vi "TEST_L1_BASELINE.vi"(5 "Serial Number":string="SN_test", 6 "error in":errorcluster, 9 "Instrument VISA in":T1={"AWG VISA"="AgilentGenerator1", "Oscilloscope  VISA "="AgilentOsciloscope", "Integration Board IP"="172.16.17.48", "connection ID"=refnum, "report out"=refnum, "report file path"=path "C:/Users/omartinez/Desktop/L0nL1_Results"}) -> (0 "error out":errorcluster, 3 "VISA Out":T1={"AWG VISA"="AgilentGenerator1", "Oscilloscope  VISA "="AgilentOsciloscope", "Integration Board IP"="172.16.17.48", "connection ID"=refnum, "report out"=refnum, "report file path"=path "C:/Users/omartinez/Desktop/L0nL1_Results"})   [LabVIEW 2012]
uses:
  <vilib>/Utility/NIReport.llb/NI_report.lvclass
  <vilib>/Utility/NIReport.llb/HTML/NI_HTML.lvclass
  <instrlib>/Agilent 8000 Series/Agilent 8000 Series.lvlib
  Sum_Abrilader/L0_Sum_Adder Folder/C/Program Files/National Instruments/LabVIEW 2012/instr.lib/Agilent 81150/Agilent 81150.lvlib
panel:
  out "Current Channel":i32=6
  in  "Combination\n  (Act High)":i32 min=0 max=127 step=1 format="%b"
  in  "Single/Comb":bool=TRUE
  in  "Single Channel Enable":i32(slide) scale=0.0..6.0
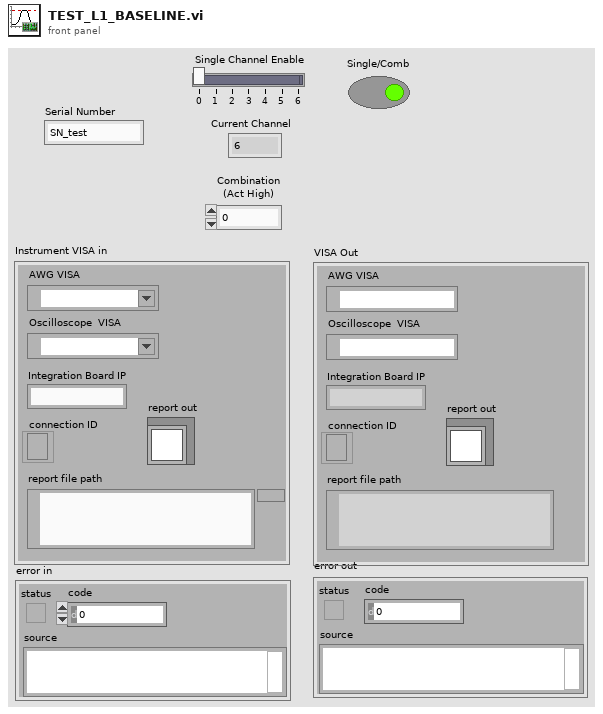
[diagram p1: front panel]
types:
  T1 = cluster{"AWG VISA":refnum<visa-resource-name>, "Oscilloscope  VISA ":refnum<visa-resource-name>, "Integration Board IP":string, "connection ID":refnum<k5>, "report out":refnum<class "NI_report.lvclass">, "report file path":path}
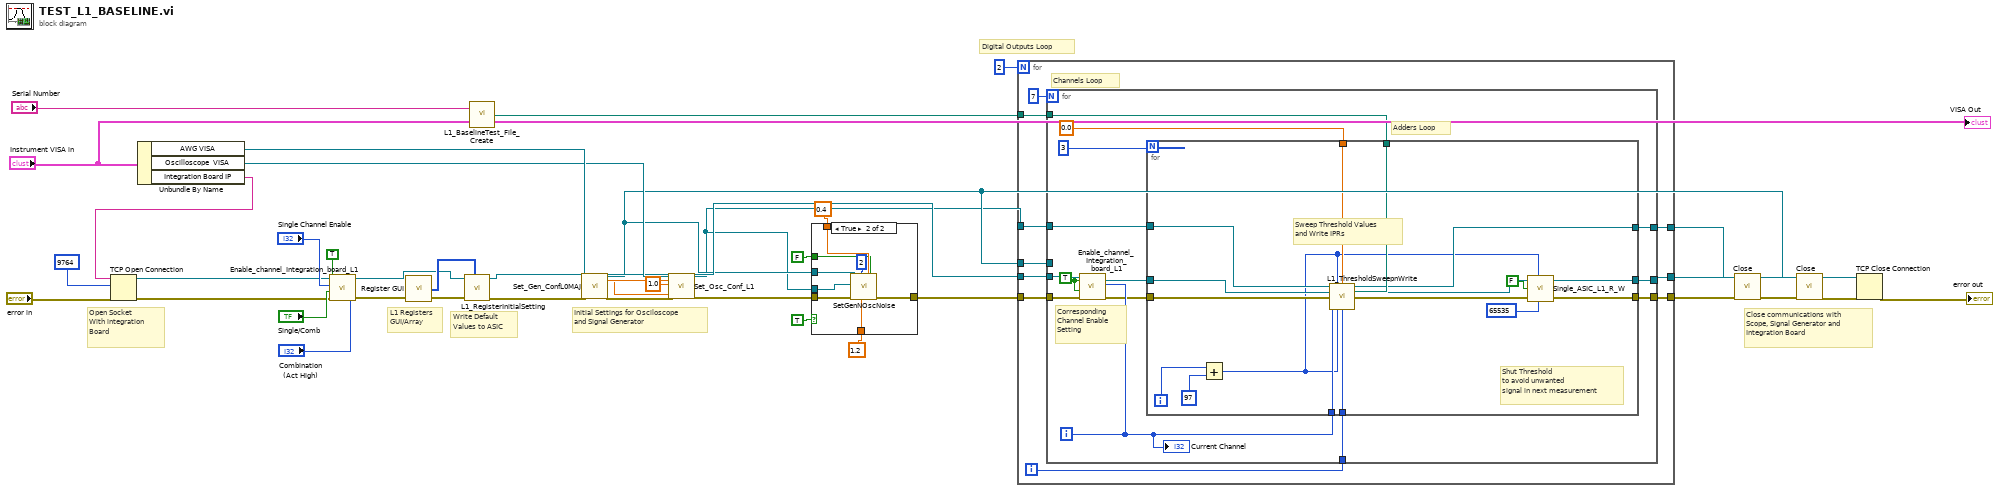
[diagram p0: block diagram]
diagram:
  # "Digital Outputs Loop"
  # "Write Default\nValues to ASIC"
  # "Close communications with \nScope, Signal Generator and \nIntegration Board"
  # "Initial Settings for Osciloscope\nand Signal Generator"
  # "L1 Registers\nGUI/Array"
  # "Open Socket\nWith integration \nBoard"
  n1 = Unbundle By Name("Instrument VISA in") -> ("AWG VISA"=w27:refnum<visa-resource-name>, "Oscilloscope  VISA"=w26:refnum<visa-resource-name>, "Integration Board IP"=w32:string)
  n2 = TCP Open Connection(address=w32, remote port or service name=9764, error in (no error)="error in") -> (connection ID=w19:refnum<k5>, error out=w10:errorcluster)  [unwired: 2 in]
  n3 = call "Enable_channel_Integration_board_L1.vi"("Combination"="Combination\n  (Act High)", "Enable  L1 single  Input"="Single Channel Enable", "error in (no error)"=w10, "SingleIN/#Combination"="Single/Comb", "Enable some/all"=TRUE ("#Enable all L1"), "connection ID"=w19) -> ("error out"=w11:errorcluster, "connection ID out"=w12:refnum<k5>)
  n4 = call "Register GUI.vi"("error in (no error)"=w11) -> ("error out"=w13:errorcluster, "REG ARRAy"=w14:u32[])  [unwired: 3 in]
  n5 = call "L1_RegisterInitialSetting.vi"("REG ARRAy"=w14, "error in"=w13, "connection ID in"=w12) -> ("error out"=w16:errorcluster, "connection ID out"=w15:refnum<k5>)  [unwired: 7 in]
  n6 = call "L1_BaselineTest_File_Create.vi"("input cluster"="Instrument VISA in", "Serial Number"="Serial Number") -> ("appended path"=w31:path)
  n7 = call "Set_Gen_ConfL0MAJ.vi"("AWG VISA"=w27, "error in (no error)"=w16) -> ("Amplitude 1 OUT"=w29:dbl, "VISA resource name out"=w4:refnum<visa-resource-name>, "Pulse Width in seconds 1 OUT"=w28:dbl, "error out"=w30:errorcluster)  [unwired: 10 in, 4 out]
  n8 = call "Set_Osc_Conf_L1.vi"("VISA resource name"=w26, "Amplitude IN"=w29, "Trigger Level IN"=1.0, "Pulse Width in seconds IN"=w28, "error in (no error)"=w30) -> ("VISA resource name out"=w3:refnum<visa-resource-name>, "error out"=w8:errorcluster)  [unwired: 13 in]
  n9 = case shown="True" TRUE {
    tunnel: [w40 w48] -> w7
    tunnel: 0.4 ("Voltage Input") -> [_ w47]
    tunnel: 1.2 ("Amp Scaler 2") -> [_ w46]
    tunnel: FALSE ("Gen Active 2") -> [_ w45]
    tunnel: w3 -> [_ w44]
    tunnel: w4 -> [_ w43]
    tunnel: w8 -> [w40 w42]
    frame False {
    }
    frame True {
      n10 = call "SetGenNOscNoise.vi"("Enable Output"=w45, "Input Voltage"=w47, "Amp Scaler"=w46, "NChannels"=2, "error in (no error)"=w42, "Oscilloscope VISA"=w44, "Generator VISA"=w43) -> ("error out 2"=w48:errorcluster)  [unwired: 4 in]
    }
  }
  n11 = for {
    N: 2 -> [_]
    tunnel: [w58] -> w33
    tunnel: w31 -> [w57]
    tunnel: [w56] -> w25
    tunnel: [w55] -> w22
    tunnel: w3 -> [w54]
    tunnel: w4 -> [w53]
    tunnel: w15 -> [w52]
    tunnel: w7 -> [w50]
    i -> [w49]
    # "Channels Loop"
    n12 = for {
      N: 7 -> [_]
      tunnel: [w72] -> w56
      tunnel: [w70] -> w58
      tunnel: w52 -> [w68]
      tunnel: w57 -> [w66]
      tunnel: w50 -> [w65]
      tunnel: w54 -> [w64]
      tunnel: [w63] -> w55
      tunnel: w53 -> [_]
      tunnel: w49 -> [w59]
      i -> [w62]
      w67 = TRUE ("#Enable all L1")
      # "Corresponding\nChannel Enable\nSetting"
      # "Adders Loop"
      n13 = call "Enable_channel_Integration_board_L1.vi"("Enable  L1 single  Input"=w62, "error in (no error)"=w65, "SingleIN/#Combination"=w67, "Enable some/all"=w67, "connection ID"=w68) -> ("error out"=w60:errorcluster, "connection ID out"=w69:refnum<k5>)  [unwired: 1 in]
      n14 = for {
        N: 3 -> [_]
        tunnel: w69 -> [w80]
        tunnel: w60 -> [w81]
        tunnel: [w88] -> w72
        tunnel: [w87] -> w70
        tunnel: w66 -> [w83]
        tunnel: w62 -> [w79]
        tunnel: 0.0 -> [w84]
        tunnel: w64 -> [w82]
        tunnel: [w76] -> w63
        tunnel: w59 -> [w74]
        i -> [w89]
        # "Sweep Threshold Values\nand Write IPRs"
        # "Shut Threshold\nto avoid unwanted\nsignal in next measurement"
        n15 = Add(x=w89, y=97) -> (x+y=w73:i32)
        n16 = call "L1_ThresholdSweepnWrite.vi"("VISA In"=w82, "Channel Register"=w73, "Vin"=w84, "File path In"=w83, "ID In"=w80, "Error In"=w81, "CH"=w79, "Active Adder"=w73, "Digital Output"=w74) -> ("VISA Out"=w76:refnum<visa-resource-name>, "ID out"=w77:refnum<k5>, "Error Out"=w78:errorcluster)  [unwired: 4 in]
        n17 = call "Single_ASIC_L1_R_W.vi"("connection ID"=w77, "Register or channel"=w73, "RD/#WR"=FALSE, "error in (no error)"=w78, "Data"=u32 65535 ("COMB DEC")) -> ("connection ID out"=w87:refnum<k5>, "error out"=w88:errorcluster)  [unwired: 1 in, 2 out]
      }
      "Current Channel" <- w62
    }
  }
  n18 = call <instrlib>:"Close.vi"("error in (no error)"=w25, "VISA resource name"=w22) -> ("error out"=w24:errorcluster)  [unwired: 9 in]
  n19 = call <instrlib>:"Close.vi"("error in (no error)"=w24, "VISA resource name"=w4) -> ("error out"=w23:errorcluster)  [unwired: 9 in]
  n20 = TCP Close Connection(connection ID=w33, error in (no error)=w23) -> (error out=→"error out":errorcluster)  [unwired: 1 in, 1 out]
  "VISA Out" <- "Instrument VISA in"
